vi "实验第二题.vi"() -> ()   [LabVIEW 2018]
panel:
  in  "input":dbl
  out "是否是素数":bool
  in  "输入":dbl
  out "累加值":dbl
  in  "成绩":dbl
  out "等级":string
  in  "?":dbl
  out "和":dbl
  out "布尔5":bool
  out "布尔4":bool
  out "布尔3":bool
  out "布尔2":bool
  out "布尔1":bool
  in  "间隔时间（ms）":dbl(slide) scale=0.0..1000.0
  in  "停止":bool
  # "第二题"
  # "第一题"
  # "第三题"
  # "第四题"
  # "第五题"
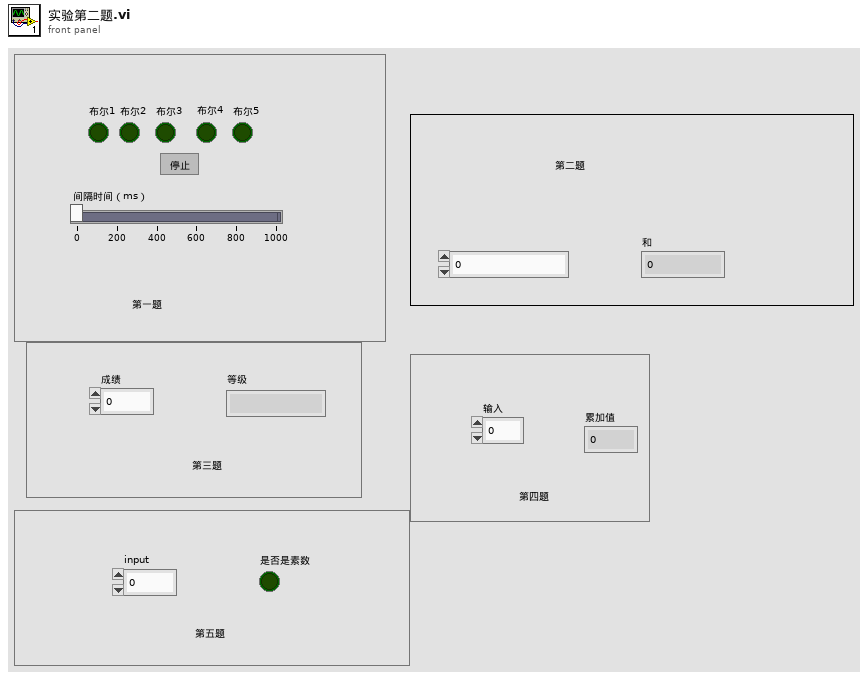
[diagram p1: front panel]
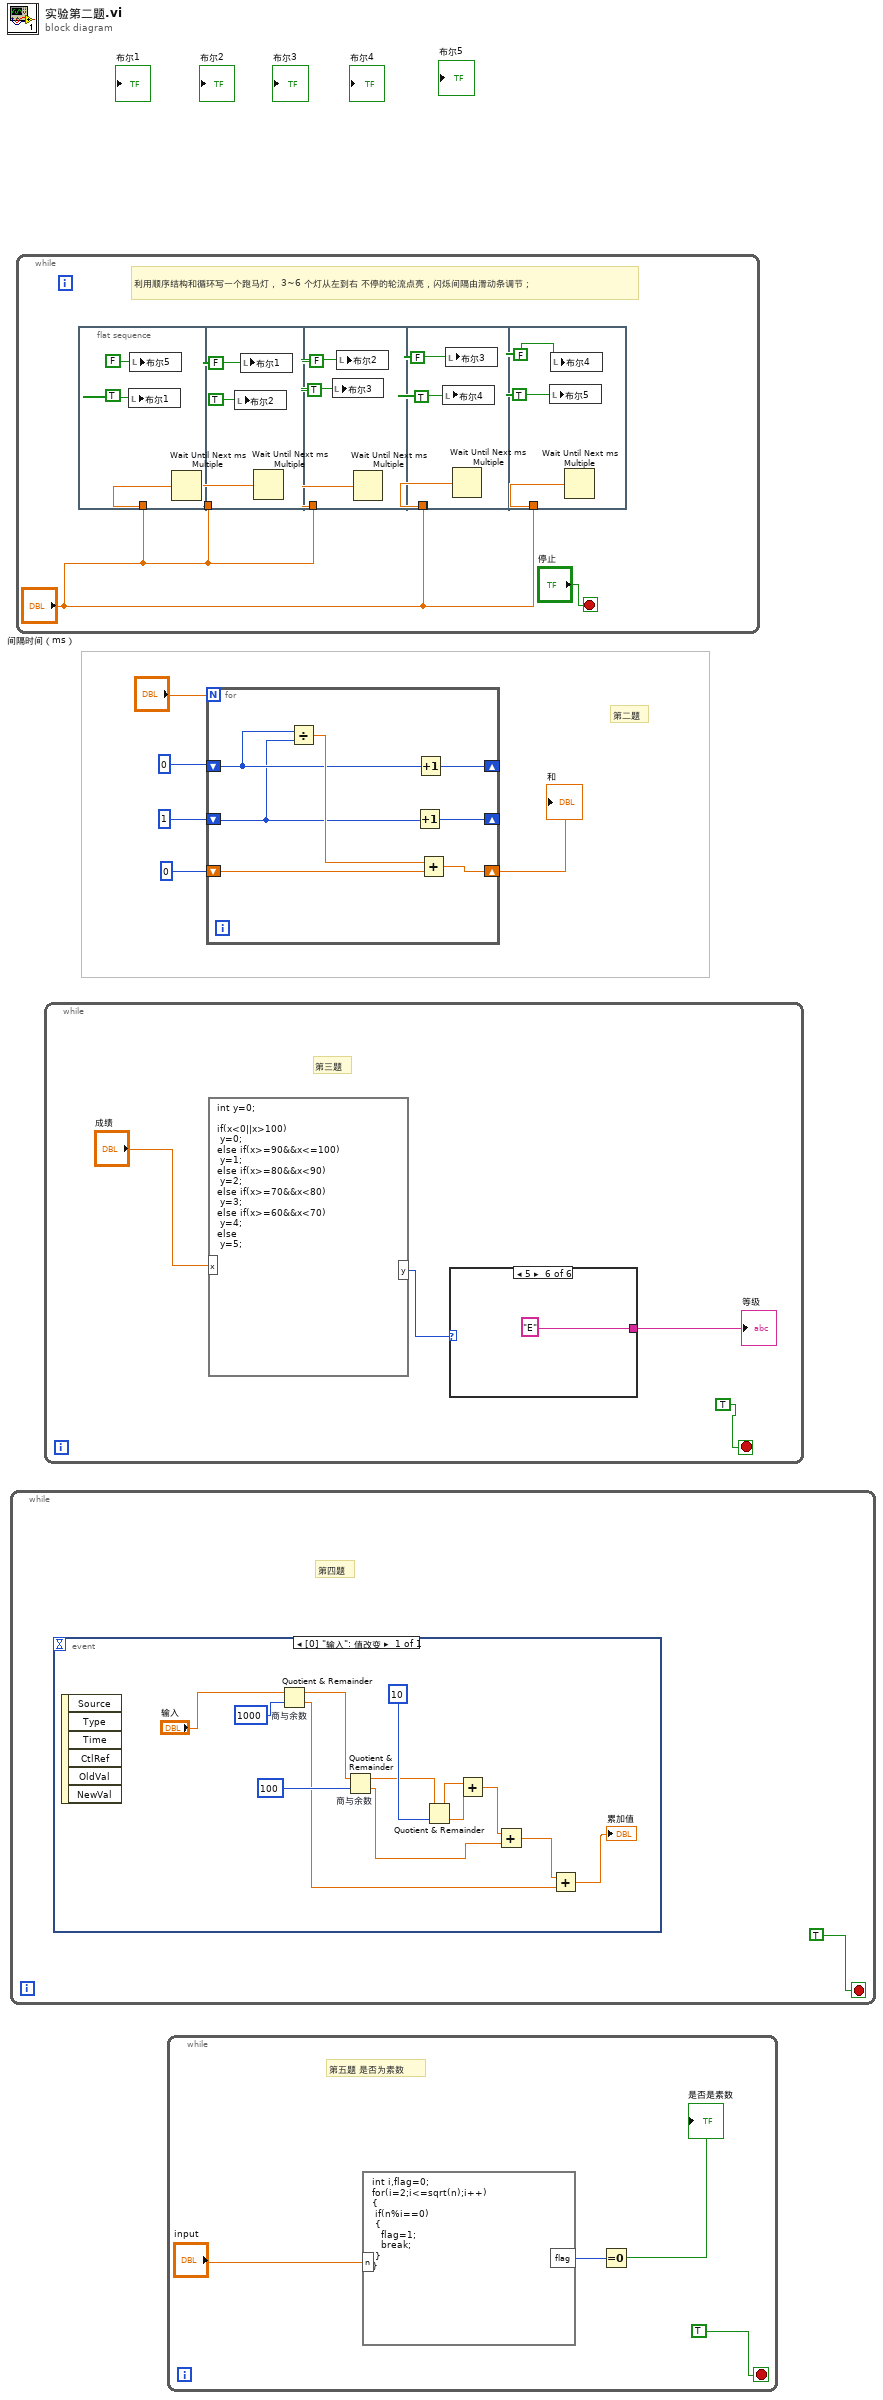
[diagram p0: block diagram]
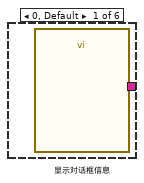
[diagram p2: hidden frame]
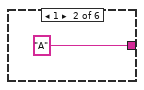
[diagram p3: hidden frame]
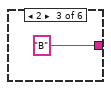
[diagram p4: hidden frame]
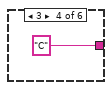
[diagram p5: hidden frame]
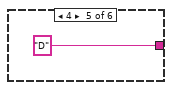
[diagram p6: hidden frame]
diagram:
  # "第二题"
  n1 = while {
    stop <- TRUE stop-if-true
    # "第四题"
  }
  n2 = while {
    stop <- "停止" stop-if-true
    # "利用顺序结构和循环写一个跑马灯， 3~6 个灯从左到右 不停的轮流点亮，闪烁间隔由滑动条调节；"
    n3 = flat-sequence {
      tunnel: "间隔时间（ms）" -> [w9]
      tunnel: "间隔时间（ms）" -> [w12]
      tunnel: "间隔时间（ms）" -> [w15]
      tunnel: [w18] -> _
      tunnel: "间隔时间（ms）" -> [w18]
      tunnel: "间隔时间（ms）" -> [w21]
      frame #0 {
        n4 = local write "布尔1"(TRUE) -> ()
        n5 = local write "布尔5"(FALSE) -> ()
        n6 = Wait Until Next ms Multiple(millisecond multiple=w9) -> ()  [unwired: 1 out]
      }
      frame #1 {
        n7 = local write "布尔2"(TRUE) -> ()
        n8 = local write "布尔1"(FALSE) -> ()
        n9 = Wait Until Next ms Multiple(millisecond multiple=w12) -> ()  [unwired: 1 out]
      }
      frame #2 {
        n10 = local write "布尔3"(TRUE) -> ()
        n11 = local write "布尔2"(FALSE) -> ()
        n12 = Wait Until Next ms Multiple(millisecond multiple=w15) -> ()  [unwired: 1 out]
      }
      frame #3 {
        n13 = local write "布尔4"(TRUE) -> ()
        n14 = local write "布尔3"(FALSE) -> ()
        n15 = Wait Until Next ms Multiple(millisecond multiple=w18) -> ()  [unwired: 1 out]
      }
      frame #4 {
        n16 = local write "布尔5"(TRUE) -> ()
        n17 = local write "布尔4"(FALSE) -> ()
        n18 = Wait Until Next ms Multiple(millisecond multiple=w21) -> ()  [unwired: 1 out]
      }
    }
  }
  n19 = while {
    stop <- TRUE stop-if-true
    # "第三题"
    n20 = formula code="int y=0;\n\nif(x<0||x>100)\n y=0;\nelse if(x>=90&&x<=100)\n y=1;\nelse if(x>=80&&x<90)\n y=2;\nelse if(x>=70&&x<80)\n y=3;\nelse if(x>=60&&x<70)\n y=4;\nelse\n y=5;"("x"="成绩") -> ("y"=w25:i32)
    n21 = case shown="5" w25 {
      tunnel: [_ "A" "B" "C" "D" "E"] -> w24
      frame 0, Default {
        n22 = call "显示对话框信息"() -> ()  [unwired: 10 in, 2 out]
      }
      frame 1 {
      }
      frame 2 {
      }
      frame 3 {
      }
      frame 4 {
      }
      frame 5 {
      }
    }
    "等级" <- w24
  }
  n23 = event shown="[0] \"输入\": 值改变" {
    selector: _ -> [_]
    dyn-events: _ -> [_]
    timeout: _ -> [_]
    event "输入": Value Change {
      n24 = event-data() -> ()  [unwired: 1 in, 6 out]
      n25 = Quotient & Remainder "商与余数"(x="输入", y=1000) -> (x-y*floor(x/y)=w36:dbl, floor(x/y)=w34:dbl)
      n26 = Quotient & Remainder "商与余数"(x=w36, y=100) -> (x-y*floor(x/y)=w42:dbl, floor(x/y)=w44:dbl)
      n27 = Quotient & Remainder(x=w42, y=10) -> (x-y*floor(x/y)=w41:dbl, floor(x/y)=w40:dbl)
      n28 = Add(x=w41, y=w40) -> (x+y=w39:dbl)
      n29 = Add(x=w39, y=w44) -> (x+y=w35:dbl)
      n30 = Add(x=w35, y=w34) -> (x+y=→"累加值":dbl)
    }
  }
  n31 = while {
    stop <- TRUE stop-if-true
    # "第五题 是否为素数"
    n32 = formula code="int i,flag=0;\nfor(i=2;i<=sqrt(n);i++)\n{\n if(n%i==0)\n {\n   flag=1;\n   break;\n }\n}"("n"="input") -> ("flag"=w48:i32)
    n33 = Equal To 0?(x=w48) -> (x = 0?=→"是否是素数":bool)
  }
  n34 = for {
    N: "?" -> [_]
    shift-right: [w56] -> _
    shift-left: 0 -> [w52]
    shift-right: [w50] -> _
    shift-left: 1 -> [w51]
    shift-right: [w53] -> w2
    shift-left: 0 -> [w54]
    n35 = Divide(x=w52, y=w51) -> (x/y=w55:dbl)
    n36 = Increment(x=w51) -> (x+1=w50:i32)
    n37 = Increment(x=w52) -> (x+1=w56:i32)
    n38 = Add(x=w55, y=w54) -> (x+y=w53:dbl)
  }
  "和" <- w2
